vi "RSI Mods to InOutMixed Mods.vi"(11 "RSI Modules in":T1[](array[typedef]) {"Module Config Data"."Config Block Data Refs"."Data Reference" format="%.0x"; "CDOutput Data"."BD Refs"."Data Reference" format="%.0x"; "CDInput Data"."BD Refs"."Data Reference" format="%.0x"; "VS ref" format="%.0x"}) -> (0 "MixedIO Mod Size Idxs":T12, 1 "Output Modules":i32[](array[numeric]), 2 "Input Mod Size Idxs":T12)   [LabVIEW 2016, in "Scan Engine Custom Device.lvlib"]
uses:
  Scan Engine Custom Device.lvlib
  Type Defs/Mod Size Indexes.ctl
  <vilib>/NI Veristand/Custom Device API/Custom Device Item Ref.ctl
  <vilib>/NI Veristand/Custom Device API/Custom Device API.lvlib
  <vilib>/NI Veristand/Custom Device API/Data Reference.ctl
  <vilib>/NI Veristand/Custom Device API/Block Data Reference.ctl
  Type Defs/Input Data.ctl
  Type Defs/Output Data.ctl
  Modules.lvlibp/RSI Module/Channel Type.ctl
  Modules.lvlibp/RSI Module/RSI Module.lvclass
  Modules.lvlibp/RSI Module/Module Models.ctl
  Type Defs/Module Config Data.ctl
  Type Defs/Mixed IO.ctl
  Type Defs/Open Module IOVs.ctl
  Type Defs/RSI Module Data.ctl
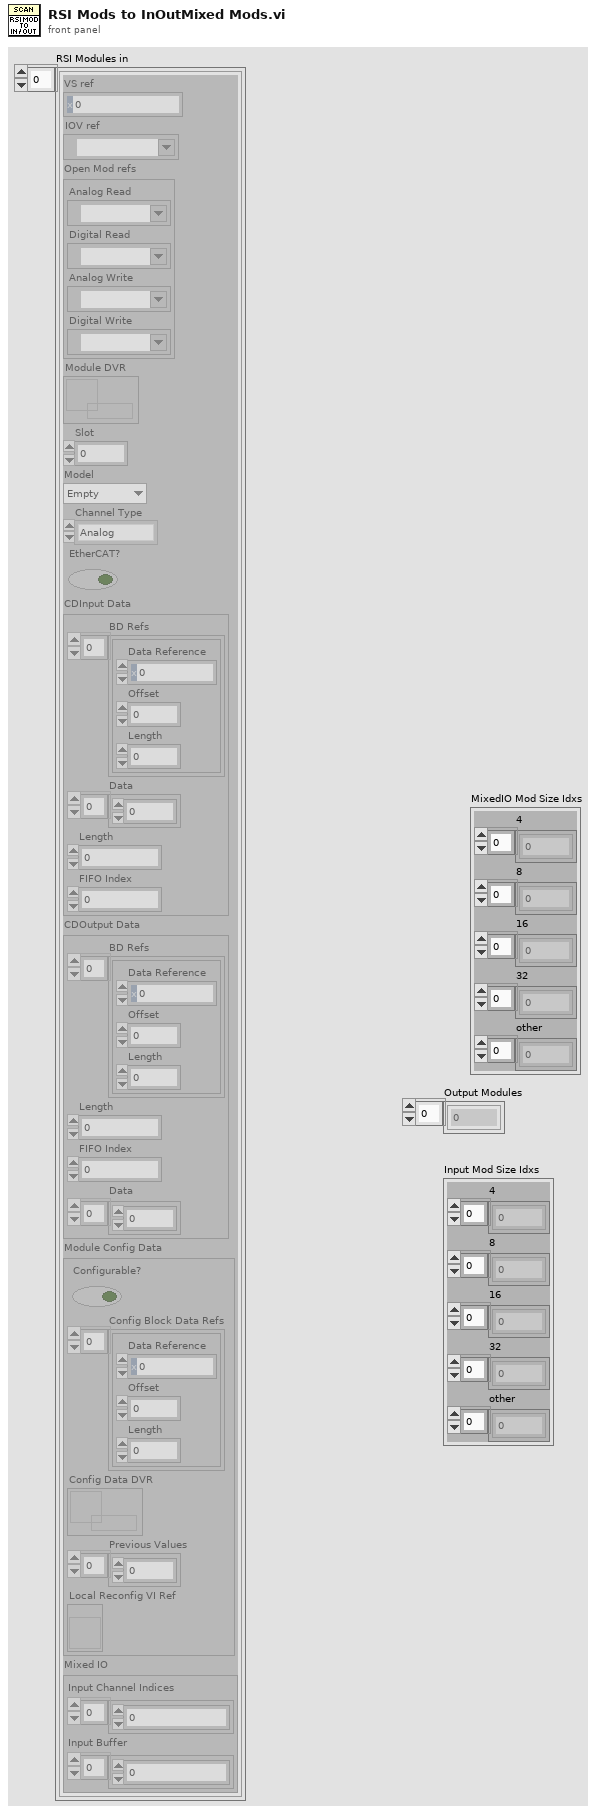
[diagram p1: front panel]
types:
  T1 = typedef "Scan Engine Custom Device.lvlib/RSI Module Data.ctl" = cluster{"VS ref":T2, "IOV ref":refnum<k21>, "Open Mod refs":T3, "Module DVR":refnum<data-value>, "Slot":u32, "Model":T4, "Channel Type":T5, "EtherCAT?":bool, "CDInput Data":T6, "CDOutput Data":T9, "Module Config Data":T10, "Mixed IO":T11}
  T2 = typedef "Custom Device API.lvlib/Custom Device Item Ref.ctl" = u64
  T3 = typedef "Scan Engine Custom Device.lvlib/Open Module IOVs.ctl" = cluster{"Analog Read":refnum<k21>, "Digital Read":refnum<k21>, "Analog Write":refnum<k21>, "Digital Write":refnum<k21>}
  T4 = typedef "Modules.lvlibp/RSI Module.lvclass/Module Models.ctl" = enum16{"Empty", "NI 9201", "NI 9203", "NI 9205", "NI 9206", "NI 9207", "NI 9208", "NI 9211", "NI 9213", "NI 9214", "NI 9215", "NI 9217", "NI 9219", "NI 9221", "NI 9225", "NI 9227", "NI 9229", "NI 9233", "NI 9234", "NI 9235", "NI 9236", "NI 9237", "NI 9239", "NI 9263", "NI 9264", "NI 9265", "NI 9269", "NI 9375", "NI 9401", "NI 9402", "NI 9403", "NI 9411", "NI 9421", "NI 9422", "NI 9423", "NI 9425", "NI 9426", "NI 9435", "NI 9472", "NI 9474", "NI 9475", "NI 9476", "NI 9477", "NI 9478", "NI 9481", "NI 9482", "NI 9485"}
  T5 = typedef "Modules.lvlibp/RSI Module.lvclass/Channel Type.ctl" = enum16{"Analog", "Digital"}
  T6 = typedef "Scan Engine Custom Device.lvlib/Input Data.ctl" = cluster{"BD Refs":T7[], "Data":dbl[], "Length":i32, "FIFO Index":i32}
  T7 = typedef "Custom Device API.lvlib/Block Data Reference.ctl" = cluster{"Data Reference":T8, "Offset":u64, "Length":u64}
  T8 = typedef "Custom Device API.lvlib/Data Reference.ctl" = i32
  T9 = typedef "Scan Engine Custom Device.lvlib/Output Data.ctl" = cluster{"BD Refs":T7[], "Length":i32, "FIFO Index":i32, "Data":dbl[]}
  T10 = typedef "Scan Engine Custom Device.lvlib/Module Config Data.ctl" = cluster{"Configurable?":bool, "Config Block Data Refs":T7[], "Config Data DVR":refnum<data-value>, "Previous Values":dbl[], "Local Reconfig VI Ref":refnum<vi>}
  T11 = typedef "Scan Engine Custom Device.lvlib/Mixed IO.ctl" = cluster{"Input Channel Indices":i32[], "Input Buffer":dbl[]}
  T12 = typedef "Scan Engine Custom Device.lvlib/Mod Size Indexes.ctl" = cluster{"4":i32[], "8":i32[], "16":i32[], "32":i32[], "other":i32[]}
  T13 = typedef "Scan Engine Custom Device.lvlib/Module IO Type.ctl" = enum16{"Input", "Output", "Mixed"}
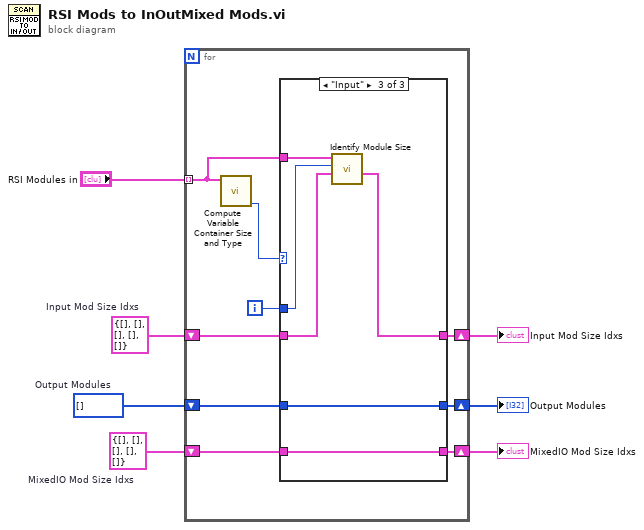
[diagram p0: block diagram]
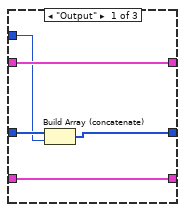
[diagram p2: hidden frame]
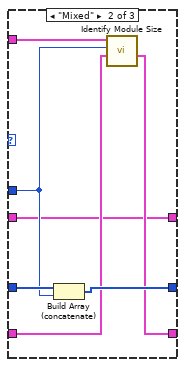
[diagram p3: hidden frame]
diagram:
  w2 = T12 {"4"=[], "8"=[], "16"=[], "32"=[], "other"=[]}  # Input Mod Size Idxs
  w4 = T12 {"4"=[], "8"=[], "16"=[], "32"=[], "other"=[]}  # MixedIO Mod Size Idxs
  w3 = i32[] []  # Output Modules
  n1 = for {
    tunnel: "RSI Modules in" -> [w8] mode=indexing
    shift-right: [w14] -> w5
    shift-left: w2 -> [w13]
    shift-right: [w16] -> w6
    shift-left: w3 -> [w15]
    shift-right: [w10] -> w7
    shift-left: w4 -> [w11]
    i -> [w9]
    n2 = call "Compute Variable Container Size and Type.vi"("RSI Module in"=w8) -> ("ModIOType"=w12:T13)  [unwired: 8 in, 2 out]
    n3 = case shown="\"Input\"" w12 {
      tunnel: [w19 w27 w34] -> w16
      tunnel: w15 -> [w21 w28 w34]
      tunnel: [w20 w22 w29] -> w14
      tunnel: w13 -> [w20 w22 w30]
      tunnel: w9 -> [w18 w24 w31]
      tunnel: w11 -> [w17 w25 w33]
      tunnel: [w17 w23 w33] -> w10
      tunnel: w8 -> [_ w26 w32]
      frame "Output" {
        n4 = Build Array (concatenate)(w21, w18) -> (w19:i32[])
      }
      frame "Mixed" {
        n5 = Build Array (concatenate)(w28, w24) -> (w27:i32[])
        n6 = call "Identify Module Size.vi"("Mod Size Idxs in"=w25, "Idx"=w24, "RSI Module"=w26) -> ("Mod Size Idxs out"=w23:T12)  [unwired: 8 in]
      }
      frame "Input" {
        n7 = call "Identify Module Size.vi"("Mod Size Idxs in"=w30, "Idx"=w31, "RSI Module"=w32) -> ("Mod Size Idxs out"=w29:T12)  [unwired: 8 in]
      }
    }
  }
  "MixedIO Mod Size Idxs" <- w7
  "Output Modules" <- w6
  "Input Mod Size Idxs" <- w5
